vi "Insert Data Point.vi"(4 "Error In":errorcluster, 7 "Data":dbl format="%.6g") -> (0 "Error Out":errorcluster)   [LabVIEW 2015, in "Sine Signal Data Buffer.lvlib"]
uses:
  Sine Signal Data Buffer.lvlib
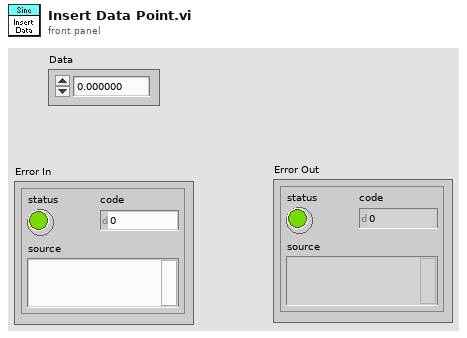
[diagram p1: front panel]
types:
  T1 = typedef "Sine Signal Data Buffer.lvlib/buffer data typedef.ctl" = cluster{"Sine Data":dbl[], "Counter":i32}
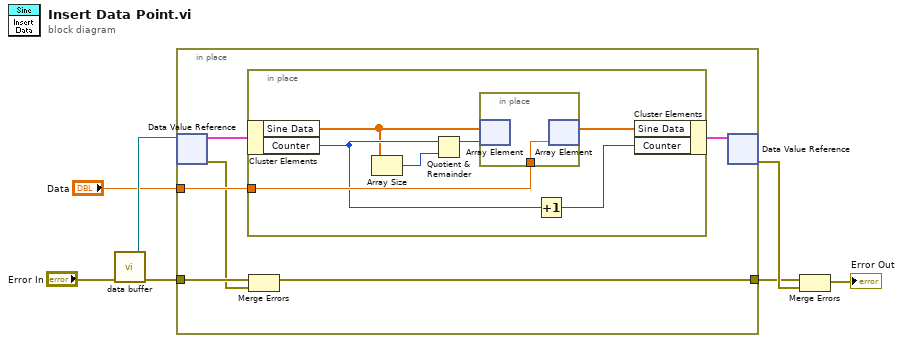
[diagram p0: block diagram]
diagram:
  n1 = call "data buffer.vi"("Error In"="Error In") -> ("Error Out"=w2:errorcluster, "DVR"=w6:refnum<data-value>)  [unwired: 5 in]
  n2 = in-place {
    in-place-border: "Data" -> [w11]
    in-place-border: w2 -> [w10]
    in-place-border: [w8] -> w1
    n3 = in-place-dvr #1(w6) -> (w13:T1, w9:errorcluster)
    n4 = in-place {
      in-place-border: w11 -> [w20]
      n5 = in-place-cluster #2(w13) -> ("Sine Data"=w15:dbl[], "Counter"=w17:i32)
      n6 = Array Size(array=w15) -> (size(s)=w14:i32)
      n7 = Quotient & Remainder(x=w17, y=w14) -> (x-y*floor(x/y)=w18:i32)  [unwired: 1 out]
      n8 = in-place {
        in-place-border: w20 -> [w21]
        n9 = in-place-array #3(w15, w18) -> ()  [unwired: 1 out]
        n10 = in-place-array #3(w21) -> (w19:dbl[])  [unwired: 1 out]
      }
      n11 = Increment(x=w17) -> (x+1=w16:i32)
      n12 = in-place-cluster #2("Sine Data"=w19, "Counter"=w16) -> (w12:T1)
    }
    n13 = Merge Errors(w10, w9) -> (w8:errorcluster)
    n14 = in-place-dvr #1(w12) -> (w3:errorcluster)  [unwired: 1 out]
  }
  n15 = Merge Errors(w1, w3) -> (→"Error Out":errorcluster)
